vi "send_enter_ch.vi"(10 "Input buffer size":u32=4096, 11 "USB Interface Name":refnum<visa-resource-name>="COM3") -> (3 "USB Interface Name out":string)   [LabVIEW 2012]
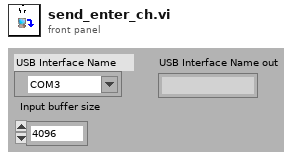
[diagram p1: front panel]
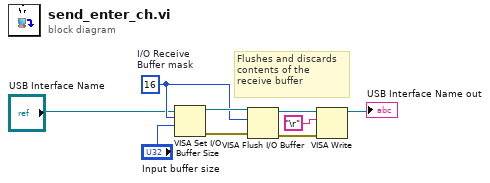
[diagram p0: block diagram]
diagram:
  w4 = u16 16  # I/O Receive Buffer mask
  # "Flushes and discards \ncontents of the \nreceive buffer"
  n1 = VISA Set I/O Buffer Size(VISA resource name="USB Interface Name", mask (16)=w4, size (4096)="Input buffer size") -> (VISA resource name out=w6:refnum<visa-resource-name>, error out=w5:errorcluster)  [unwired: 1 in]
  n2 = VISA Flush I/O Buffer(VISA resource name=w6, mask (16)=w4, error in (no error)=w5) -> (VISA resource name out=w9:refnum<visa-resource-name>, error out=w8:errorcluster)
  n3 = VISA Write(VISA resource name=w9, write buffer="\r", error in (no error)=w8) -> (VISA resource name out=→"USB Interface Name out":refnum<visa-resource-name>)  [unwired: 2 out]
